vi "Write Image Header.vi"(8 "error in (no error)":errorcluster, 11 "CCD in":refnum<class "CCD.lvclass">) -> (0 "error out":errorcluster, 3 "CCD out":refnum<class "CCD.lvclass">)   [LabVIEW 2018, in "CCD.lvclass"]
uses:
  CCD.lvclass
  CCD.lvclass/CCD.ctl
  <userlib>/gfitsio/gfitsio-write-key-string.vi
  <userlib>/gfitsio/gfitsio.lvlib
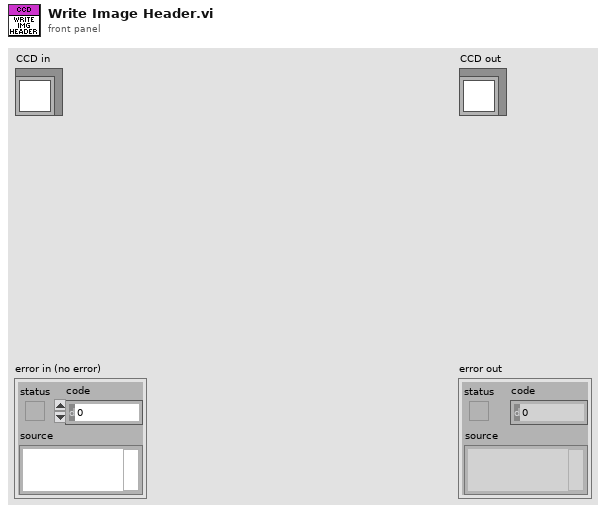
[diagram p1: front panel]
types:
  T1 = enum16{"open", "open or create", "create or replace", "create", "open (read only)"}
  T2 = typedef "gfitsio.lvlib/gfitsio-refnum.ctl" = refnum<k1>
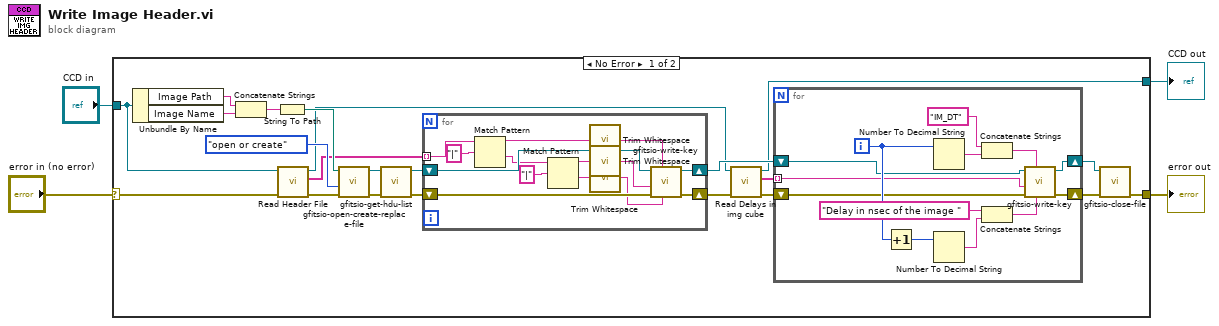
[diagram p0: block diagram]
diagram:
  n1 = case shown="No Error" "error in (no error)" {
    selector: "error in (no error)" -> [w16 w55]
    tunnel: [w21 w55] -> w2
    tunnel: [w12 w54] -> w1
    tunnel: "CCD in" -> [w14 w54]
    frame No Error {
      n2 = Unbundle By Name(w14) -> ("Image Path"=w7:string, "Image Name"=w6:string)
      n3 = Concatenate Strings(w7, w6) -> (w5:string)
      n4 = String To Path(string=w5) -> (path=w26:path)
      n5 = call "Read Header File.vi"("error in (no error)"=w16, "CCD in"=w14) -> ("error out"=w15:errorcluster, "Header Contents"=w9:string[], "CCD out"=w13:refnum<class "CCD.lvclass">)  [unwired: 7 in]
      n6 = call <userlib>:"gfitsio-open-create-replace-file.vi"("error in (no error)"=w15, "function (open)"=T1."open or create", "file path (dialog if empty)"=w26) -> ("error out"=w25:errorcluster, "gfits refnum"=w24:T2)  [unwired: 6 in, 1 out]
      n7 = call <userlib>:"gfitsio-get-hdu-list.vi"("error in (no error)"=w25, "gfits refnum"=w24) -> ("error out"=w22:errorcluster, "dup gfits refnum"=w23:T2)  [unwired: 6 in, 2 out]
      n8 = for {
        shift-right: [w53] -> w18
        shift-left: w23 -> [w51]
        shift-right: [w52] -> w11
        shift-left: w22 -> [w50]
        tunnel: w9 -> [w49] mode=indexing
        n9 = Match Pattern(string=w49, regular expression="|") -> (before substring=w41:string, after substring=w47:string)  [unwired: 1 in, 2 out]
        n10 = Match Pattern(string=w47, regular expression="|") -> (before substring=w45:string, after substring=w43:string)  [unwired: 1 in, 2 out]
        n11 = call <vilib>:"Trim Whitespace.vi"("string"=w41) -> ("trimmed string"=w40:string)  [unwired: 1 in]
        n12 = call <vilib>:"Trim Whitespace.vi"("string"=w45) -> ("trimmed string"=w44:string)  [unwired: 1 in]
        n13 = call <vilib>:"Trim Whitespace.vi"("string"=w43) -> ("trimmed string"=w42:string)  [unwired: 1 in]
        n14 = call-poly <userlib>:"gfitsio-write-key.vi"("comment"=w42, "keyname"=w40, "error in (no error)"=w50, "value"=w44, "gfits refnum"=w51) -> ("error out"=w52:errorcluster, "dup gfits refnum"=w53:T2)  [unwired: 5 in]
      }
      n15 = call "Read Delays in img cube.vi"("error in (no error)"=w11, "CCD in"=w13) -> ("error out"=w10:errorcluster, "Delays in img cube"=w8:string[], "CCD out"=w12:refnum<class "CCD.lvclass">)  [unwired: 7 in]
      n16 = for {
        shift-right: [w32] -> w19
        shift-left: w10 -> [w33]
        shift-right: [w30] -> w17
        shift-left: w18 -> [w31]
        tunnel: w8 -> [w27] mode=indexing
        i -> [w35]
        n17 = Increment(x=w35) -> (x+1=w36:i32)
        n18 = Number To Decimal String(number=w35) -> (decimal integer string=w38:string)  [unwired: 1 in]
        n19 = Number To Decimal String(number=w36) -> (decimal integer string=w28:string)  [unwired: 1 in]
        n20 = Concatenate Strings("IM_DT", w38) -> (w37:string)
        n21 = Concatenate Strings("Delay in nsec of the image " ("comment"), w28) -> (w34:string)
        n22 = call-poly <userlib>:"gfitsio-write-key.vi"("comment"=w34, "keyname"=w37, "error in (no error)"=w33, "value"=w27, "gfits refnum"=w31) -> ("error out"=w32:errorcluster, "dup gfits refnum"=w30:T2)  [unwired: 5 in]
      }
      n23 = call <userlib>:"gfitsio-close-file.vi"("error in (no error)"=w19, "gfits refnum"=w17) -> ("error out"=w21:errorcluster)  [unwired: 8 in, 1 out]
    }
    frame Error {
    }
  }
  "error out" <- w2
  "CCD out" <- w1
